vi "listen for stop or shutdown.vi"(8 "error in (no error)":errorcluster) -> (0 "error out":errorcluster, 3 "Shutdown command received?":bool)   [LabVIEW 2012, in "GFG library.lvlib"]
doc: "SciScan 1.2 160622"
uses:
  GFG/GFG library.lvlib
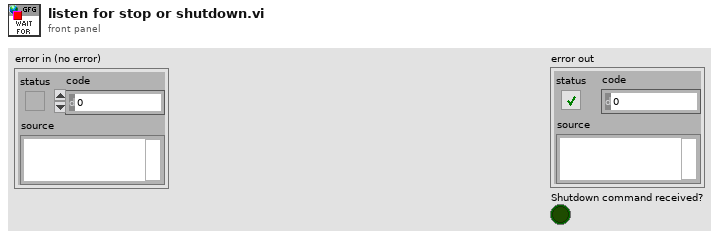
[diagram p1: front panel]
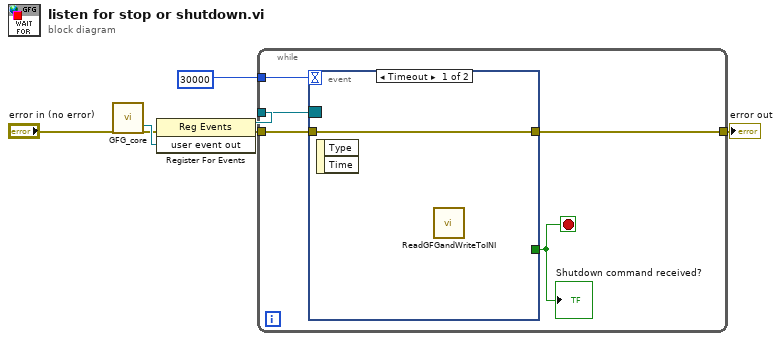
[diagram p0: block diagram]
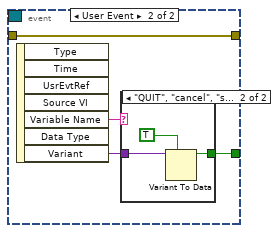
[diagram p2: hidden frame]
diagram:
  n1 = call "GFG_core.vi"("error in (no error)"="error in (no error)") -> ("user event out"=w6:refnum<user-event>, "error out"=w5:errorcluster)  [unwired: 12 in, 5 out]
  n2 = register-events(error in=w5, w6) -> (reference out=w7:refnum<event-registration>, error out=w3:errorcluster)  [unwired: 1 in]
  n3 = while {
    tunnel: w7 -> [w12]
    tunnel: w3 -> [w10]
    tunnel: [w9] -> w2
    tunnel: 30000 -> [w8]
    stop <- w11 stop-if-true
    n4 = event shown="[0] Timeout" {
      selector: w12 -> [_ _]
      dyn-events: _ -> [_ _]
      timeout: w8 -> [_ _]
      tunnel: [_ w15] -> w11
      tunnel: w10 -> [w13 w14]
      tunnel: [w13 w14] -> w9
      event Timeout {
        n5 = event-data() -> ()  [unwired: 1 in, 2 out]
        n6 = call "ReadGFGandWriteToINI.vi"() -> ()  [unwired: 11 in, 1 out]
      }
      event User Event {
        n7 = event-data() -> ("Variable Name"=w17:string, "Variant"=w16:variant)  [unwired: 1 in, 5 out]
        n8 = case shown="\"QUIT\", \"cancel\", \"shutdown\"" w17 {
          tunnel: w16 -> [_ w20]
          tunnel: [_ w18] -> w15
          frame "False", Default {
          }
          frame "QUIT", "cancel", "shutdown" {
            n9 = Variant To Data(type=TRUE ("want seconds? (F)"), Variant=w20) -> (data=w18:bool)  [unwired: 1 in, 1 out]
          }
        }
      }
    }
    "Shutdown command received?" <- w11
  }
  "error out" <- w2
